vi "Start Fan.vi"(8 "error in (no error)":errorcluster, 10 "Fan Speed":dbl, 11 "Fan Controller in":refnum<class "Fan Controller.lvclass">) -> (0 "error out":errorcluster, 3 "Fan Controller out":refnum<class "Fan Controller.lvclass">)   [LabVIEW 2019, in "Fan Controller.lvclass"]
uses:
  <vilib>/gpm_packages/@cs/Car-wash/Source/Fan Controller/Fan Controller.lvclass
  <vilib>/gpm_packages/@cs/Car-wash/Source/iFan Controller/iFan Controller.lvclass
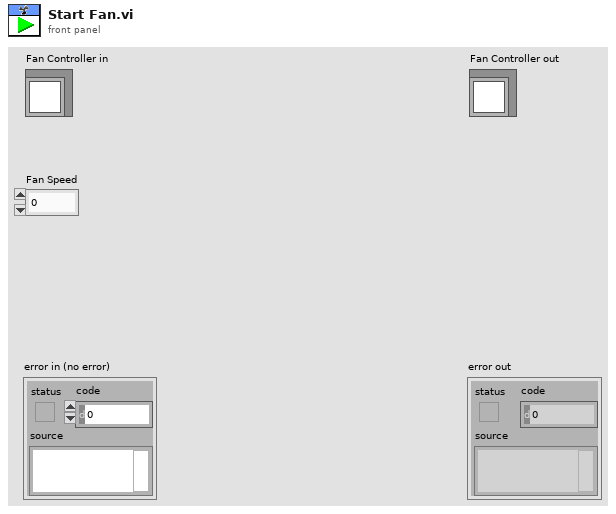
[diagram p1: front panel]
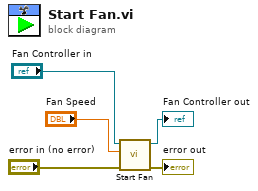
[diagram p0: block diagram]
diagram:
  n1 = call-parent "Start Fan.vi"("error in (no error)"="error in (no error)", "Fan Speed"="Fan Speed", "iFan Controller in"="Fan Controller in") -> ("error out"=→"error out":errorcluster, "iFan Controller out"=→"Fan Controller out":refnum<class "Fan Controller.lvclass">)  [unwired: 7 in]
